vi "Inficon VGC.vi"() -> ()   [LabVIEW 2015]
doc: "Example VI that demonstrates all library features."
uses:
  PL Inficon VGC.lvclass
panel:
  in  "error acknowledgement":u16(ring) items=["manual", "auto"]
  out "temperature, °C":i32
  in  "Torr lock":u16(ring) items=["off", "on"]
  in  "test keys":bool
  out "relay test relays":bool[](array[boolean])
  out "relay test state":u16(ring) items=["off", "on"]
  in  "test relays":bool
  in  "test flash":bool
  in  "test EEPROM":bool
  in  "usb flash inserted":bool
  in  "test display":bool
  in  "test ID resistance":bool
  in  "test ADC":bool
  out "operating hours":u32
  out "MAC address":string
  in  "keylock":u16(ring) items=["off", "on"]
  in  "compatibility":u16(ring) items=["Inficon gauges", "OLV transmitter"]
  in  "usb":T1 {"state" items=["loaded", "loading", "load", "format", "delete"]}
  in  "data logger":T2 {"decimal separator" items=["comma", "point"]; "interval" items=["1 s", "10 s", "30 s", "60 s", "value change >= 1 %", "value change >= 5 %"]; "action" items=["stop", "start", "clear"]}
  in  "date and time":timestamp
  out "device information":T3
  in  "parameters":u16(ring) items=["default", "user"]
  in  "save parameters":bool
  in  "pressure unit":u16(ring)=4 items=["mbar/bar", "Torr", "Pa", "uHg", "hPa", "V"]
  in  "Pirani range\nextension":u16(ring) items=["disabled", "enabled"]
  in  "error relay":u16(ring) items=["all", "unit", "sensor 1 & unit", "sensor 2 & unit", "sensor 3 & unit"]
  in  "display settings":T4 {"bar graph"."graph mode" items=["off", "full scale", "full scale, high level", "full scale, setpoint", "decade", "decade, high level", "decade setpoint", "f(t), 0.2 s/pixel", "f(t), 1 s/pixel", "f(t), 6 s/pixel", "f(t), 1 min./pixel"]; "bar graph"."channel" items=["channel 1", "channel 2", "channel 3"]; "display resolutions" items=["auto", "1 digit", "2 digits", "3 digits", "4 digits"]; "range" items=["UR/OR", "value"]; "number format" items=["floating point", "exponential"]; "language" items=["English", "German", "French"]; "screensaver" items=["off", "10 min.", "30 min.", "1 hour", "2 hours", "8 hours", "backlight off after 1 min."]; "contrast, %" scale=0.0..100.0; "backlight, %" scale=0.0..100.0}
  in  "communication settings":T5={"baud rate"=115200, "ethernet"={"dhcp"=0, "ip address"="", "subnet mask"="", "default gateway"=""}} {"ethernet"."dhcp" items=["disabled", "enabled"]; "baud rate" items=["9600"=9600, "19200"=19200, "38400"=38400, "57600"=57600, "115200"=115200]}
  in  "analog output":cluster{"channel":u16, "characteristic":u16} {"characteristic" items=["log", "log a", "log -6", "log -3", "log +0", "log +3", "log c1", "log c2", "log c3", "lin -10", "lin -9", "lin -8", "lin -7", "lin -6", "lin -5", "lin -4", "lin -3", "lin -2", "lin -1", "lin +0", "lin +1", "lin +2", "lin +3", "IM221", "log c4", "PM411", "ch x", "PRM10K", "IMR110", "IMR120", "IMR310", "IMR320"]; "channel" items=["channel 1", "channel 2", "channel 3"]}
  in  "gauge activation":T6 {"deactivation" items=["manual"=0, "self control"=1, "channel 1"=3, "channel 2"=4, "channel 3"=5]; "thresholds"."off" format="%#_5p"; "thresholds"."on" format="%#_5p"; "activation" items=["manual"=0, "hot start"=1, "channel 1"=3, "channel 2"=4, "channel 3"=5]}
  in  "gauge index":u16(ring)=1 caption="gauge" items=["1"=1, "2"=2, "3"=3]
  in  "continuous time interval":u16(ring)=1 items=["100 ms", "1 s", "1 min."]
  out "continuous read":bool
  out "continuous measurement graph":cluster{dbl, dbl, dbl[][]}(graph)
  in  "continuous measurement":bool
  in  "reset errors":bool
  in  "offset values":dbl[](array[numeric])
  in  "offset modes":u16[](array[ring]) items=["off", "on", "auto", "zero"]
  in  "HV":u16[](array[ring]) items=["off", "on"]
  in  "gas correction":u16[](array[ring]) items=["nitrogen/air", "argon", "hydrogen", "helium", "neon", "krypton", "xenon", "other"]
  in  "ranges":u16[](array[ring]) items=["0.01 mbar", "0.01 Torr", "0.02 mbar", "0.02 Torr", "0.05 mbar", "0.05 Torr", "0.1 mbar", "0.1 Torr", "0.25 mbar", "0.25 Torr", "0.5 mbar", "0.5 Torr", "1 mbar", "1 Torr", "2 mbar", "2 Torr", "5 mbar", "5 Torr", "10 mbar", "10 Torr", "20 mbar", "20 Torr", "50 mbar", "50 Torr", "100 mbar", "100 Torr", "200 mbar", "200 Torr", "500 mbar", "500 Torr", "1000 mbar", "1100 mbar", "1000 Torr", "2 bar", "5 bar", "10 bar", "50 bar"]
  in  "filters":u16[](array[ring]) items=["off", "fast", "normal", "slow"]
  in  "filaments":u16[](array[ring]) items=["auto", "filament 1", "filament 2"]
  in  "emissions":u16[](array[ring]) items=["manual", "auto"]
  in  "degas":u16[](array[ring]) items=["off", "on"]
  in  "calibration factors":dbl[](array[numeric]) format="%#.3g"
  in  "switching function index":u16(ring)=1 caption="switching function" items=["1"=1, "2"=2, "3"=3, "4"=4, "5"=5, "6"=6]
  in  "switching function":T7={"mode"=1, "thresholds"={"lower"=0.0, "upper"=0.0}, "on"=FALSE} {"thresholds"."upper" format="%#_5p"; "thresholds"."lower" format="%#_5p"; "mode" items=["off", "on", "channel 1", "channel 2", "channel 3"]}
  out "gauges":T8(array[cluster]) {"status" items=["data ok", "underrange", "overrange", "sensor error", "sensor off", "no sensor", "identification error", "error BPG, HPG, BCG"]; "value" format="%#_4p"}
  out "combined measured value":dbl
  in  "combined measurement channels":u16[](array[ring]) items=["no gauge", "channel 1", "channel 2", "channel 3"]
  out "error status":T9
  out "VGC":refnum<class "PL Inficon VGC.lvclass">
  in  "interface":enum32{"serial", "TCP"}(tab)
  in  "serial settings":T10={"port"="", "baud rate"=115200} {"baud rate" items=["9600"=9600, "19200"=19200, "38400"=38400, "57600"=57600, "115200"=115200]}
  in  "TCP settings":cluster{"ip address":string, "port":u16}={"ip address"="192.168.1.1", "port"=8000}
  out "error":errorcluster
  in  "stop":bool
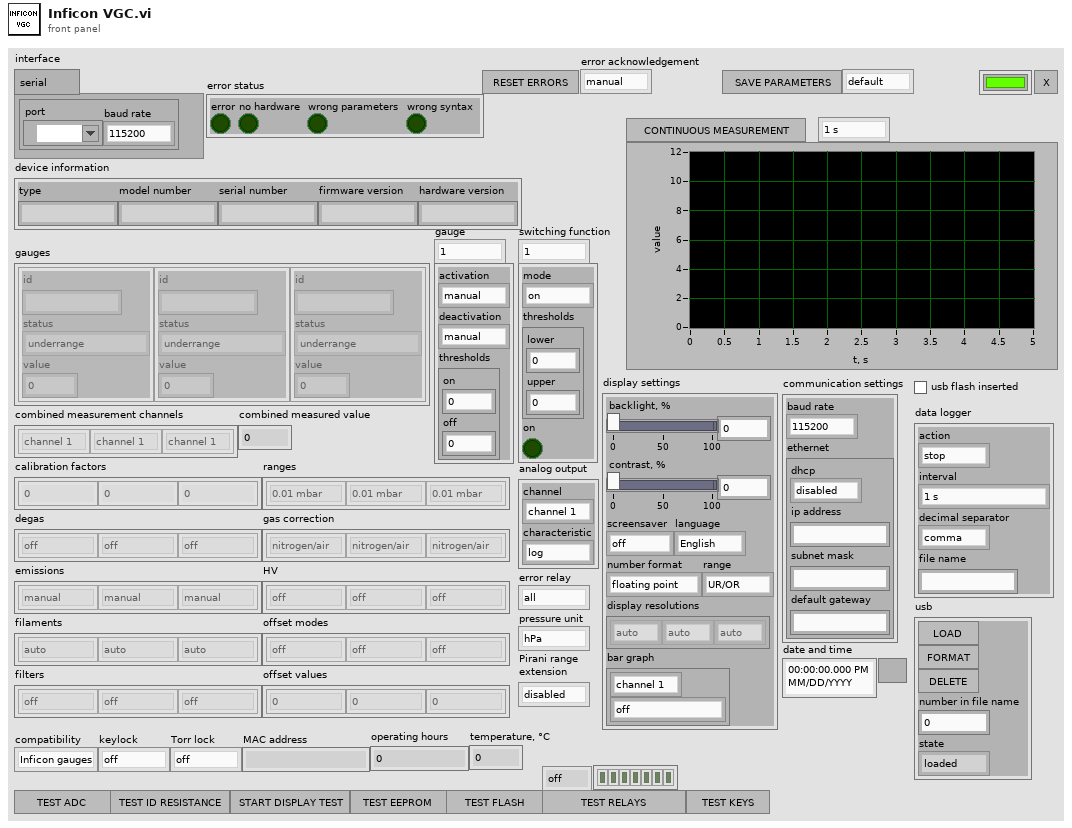
[diagram p1: front panel]
types:
  T1 = cluster{"load":bool, "format":bool, "delete":bool, "number in file name":u8, "state":u16}
  T2 = cluster{"action":u16, "interval":u16, "decimal separator":u16, "file name":string}
  T3 = cluster{"type":string, "model number":string, "serial number":string, "firmware version":string, "hardware version":string}
  T4 = cluster{"backlight, %":u8, "contrast, %":u8, "screensaver":u16, "language":u16, "number format":u16, "range":u16, "display resolutions":u16[], "bar graph":cluster{"channel":u16, "graph mode":u16}}
  T5 = cluster{"baud rate":u32, "ethernet":cluster{"dhcp":u32, "ip address":string, "subnet mask":string, "default gateway":string}}
  T6 = cluster{"activation":u16, "deactivation":u16, "thresholds":cluster{"on":dbl, "off":dbl}}
  T7 = cluster{"mode":u16, "thresholds":cluster{"lower":dbl, "upper":dbl}, "on":bool}
  T8 = cluster{"id":string, "status":u16, "value":dbl}[]
  T9 = cluster{"error":bool, "no hardware":bool, "wrong parameters":bool, "wrong syntax":bool}
  T10 = cluster{"port":refnum<visa-resource-name>, "baud rate":u32}
  T11 = cluster{"switching function relay 1":bool, "switching function relay 2":bool, "switching function relay 3":bool, "switching function relay 4":bool, "switching function relay 5":bool, "switching function relay 6":bool, "error relay":bool}
  T12 = cluster{"String":string, "status":u16, "value":dbl}
  T13 = cluster{"Boolean array[0]":bool, "Boolean array[1]":bool, "Boolean array[2]":bool, "Boolean array[3]":bool, "Boolean array[4]":bool, "Boolean array[5]":bool, "Boolean array[6]":bool}
  T14 = cluster{"key 1":u16, "key 2":u16, "key 3":u16, "key 4":u16}
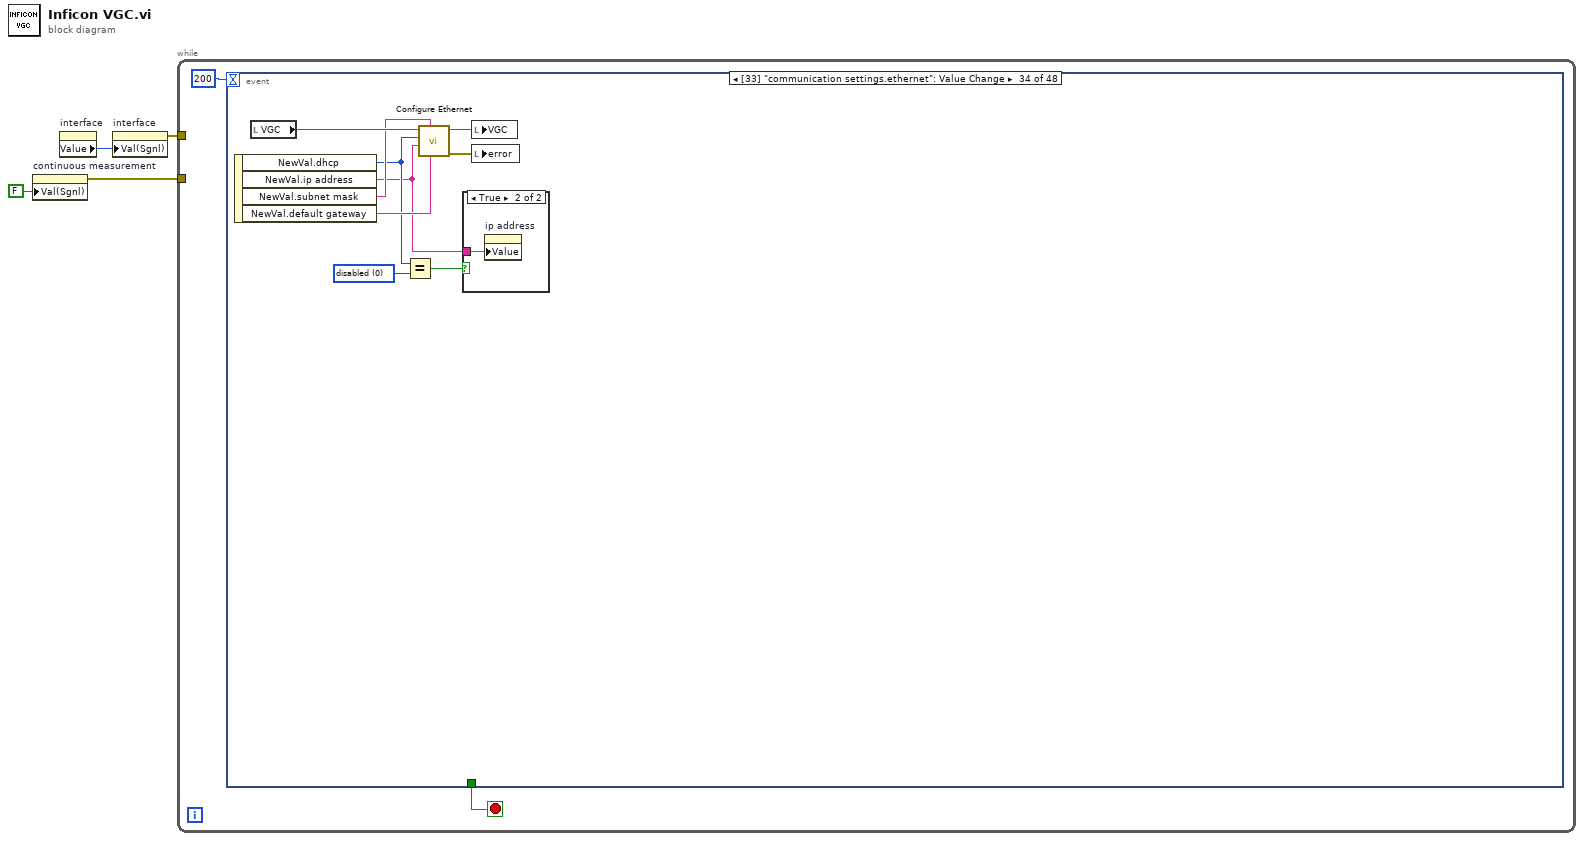
[diagram p0: block diagram]
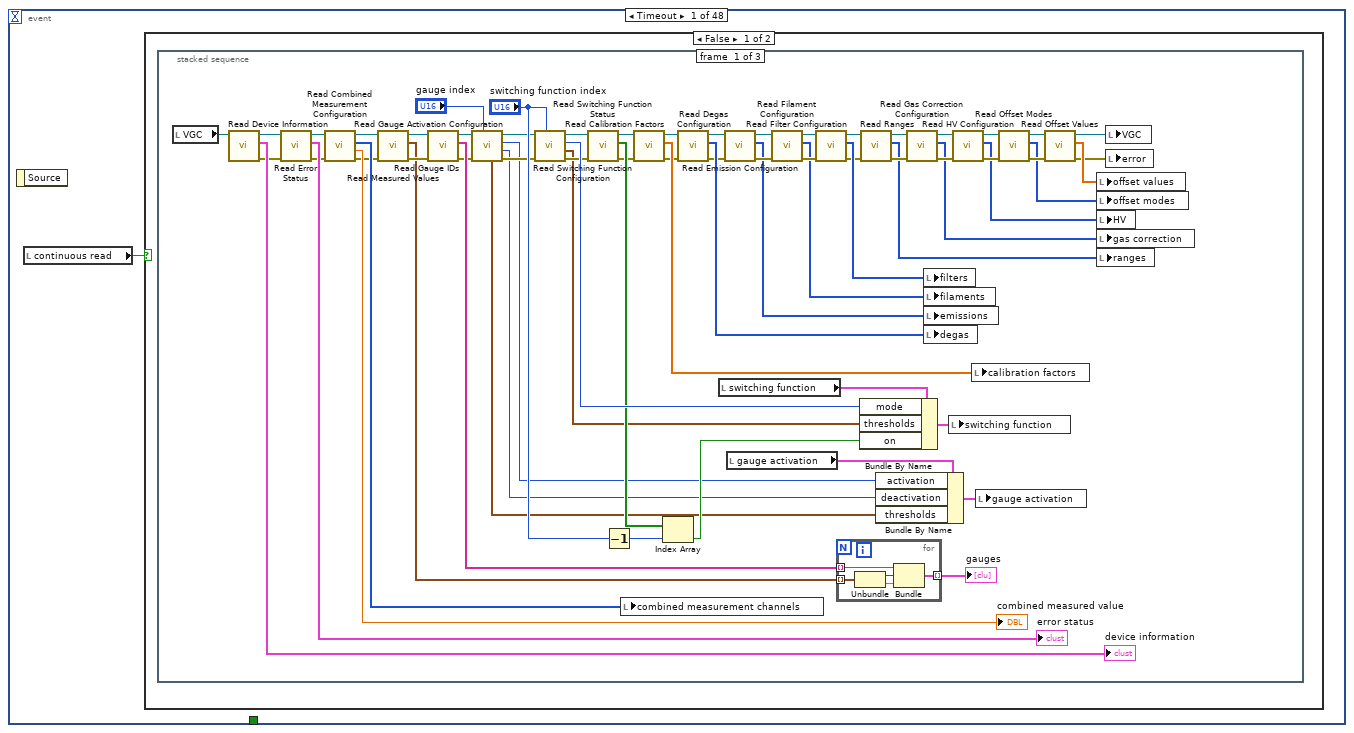
[diagram p2: hidden frame]
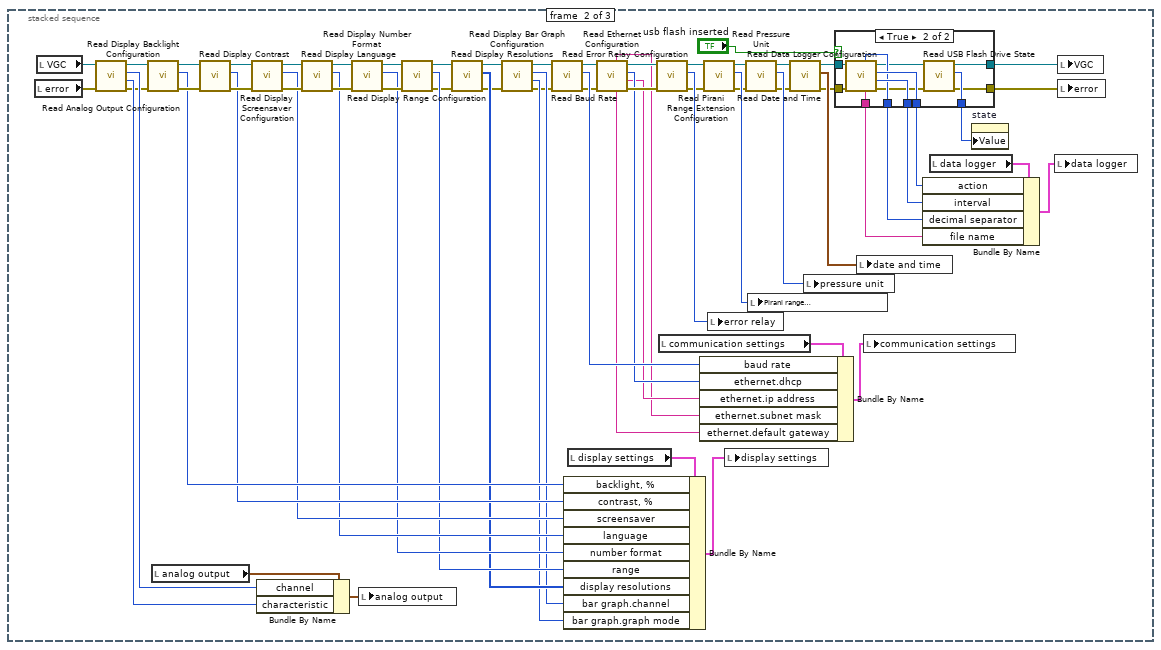
[diagram p3: hidden frame]
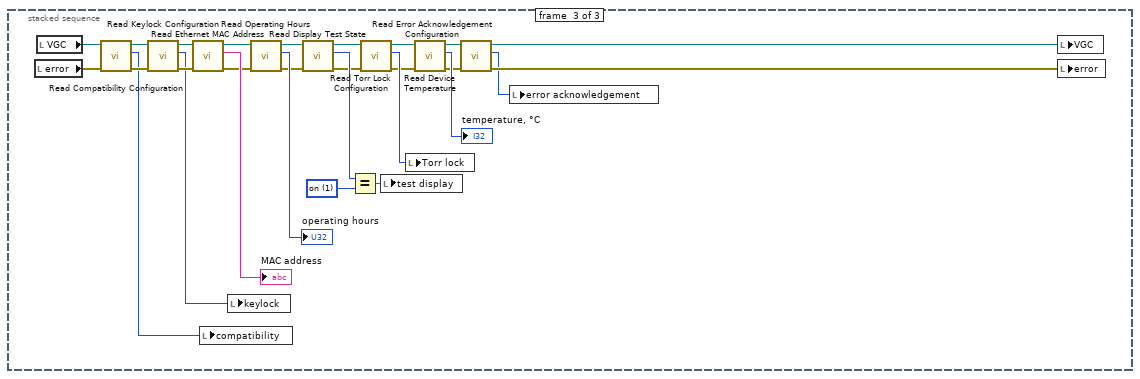
[diagram p5: hidden frame]
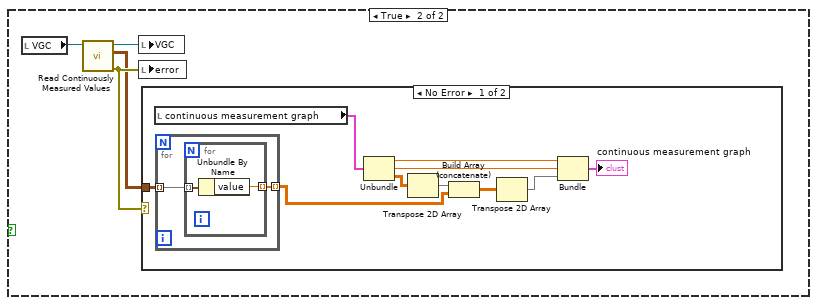
[diagram p6: hidden frame]
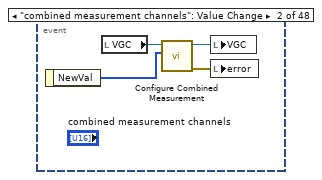
[diagram p8: hidden frame]
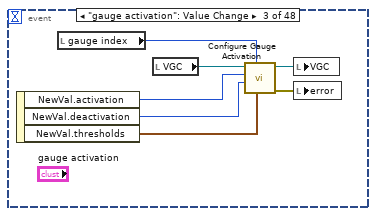
[diagram p9: hidden frame]
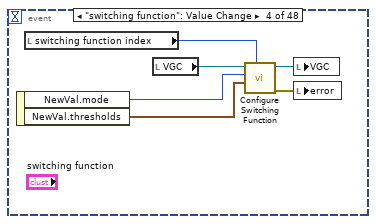
[diagram p10: hidden frame]
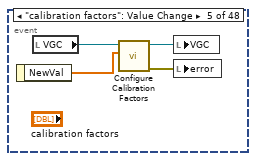
[diagram p11: hidden frame]
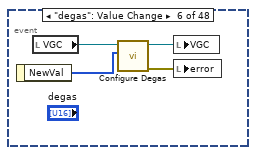
[diagram p12: hidden frame]
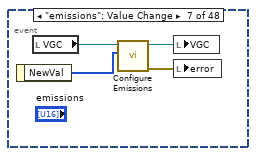
[diagram p13: hidden frame]
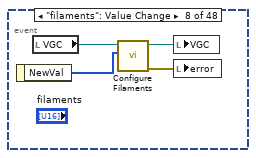
[diagram p14: hidden frame]
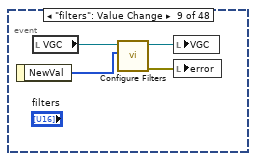
[diagram p15: hidden frame]
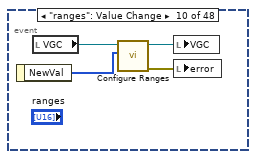
[diagram p16: hidden frame]
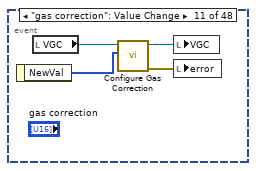
[diagram p17: hidden frame]
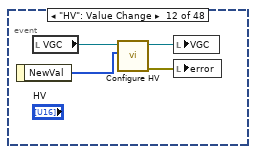
[diagram p18: hidden frame]
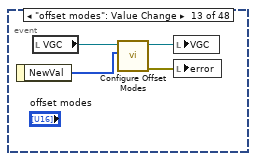
[diagram p19: hidden frame]
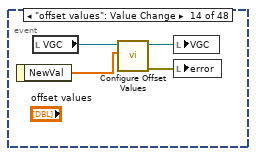
[diagram p20: hidden frame]
diagram:
  n1 = property on="continuous measurement" class="Bool (strict)"("Val(Sgnl)"=FALSE ("Value (Signaling)")) -> (error out=w1:errorcluster)  [unwired: 2 in, 1 out]
  n2 = property on="interface" class="TabCtl (strict)"() -> ("Value"=w4:enum32{"serial", "TCP"})  [unwired: 2 in, 2 out]
  n3 = property on="interface" class="TabCtl (strict)"("Val(Sgnl)"=w4) -> (error out=w3:errorcluster)  [unwired: 2 in, 1 out]
  n4 = while {
    tunnel: w3 -> [_]
    tunnel: w1 -> [_]
    stop <- w5 stop-if-true
    n5 = event shown="[33] \"communication settings.ethernet\": Value Change" {
      selector: _ -> [_ _ _ _ _ _ _ _ _ _ _ _ _ _ _ _ _ _ _ _ _ _ _ _ _ _ _ _ _ _ _ _ _ _ _ _ _ _ _ _ _ _ _ _ _ _ _ _]
      dyn-events: _ -> [_ _ _ _ _ _ _ _ _ _ _ _ _ _ _ _ _ _ _ _ _ _ _ _ _ _ _ _ _ _ _ _ _ _ _ _ _ _ _ _ _ _ _ _ _ _ _ _]
      timeout: 200 -> [_ _ _ _ _ _ _ _ _ _ _ _ _ _ _ _ _ _ _ _ _ _ _ _ _ _ _ _ _ _ _ _ _ _ _ _ _ _ _ _ _ _ _ _ _ _ _ _]
      tunnel: [_ _ _ _ _ _ _ _ _ _ _ _ _ _ _ _ _ _ _ _ _ _ _ _ _ _ _ _ _ _ _ _ _ _ _ _ _ _ _ _ _ _ _ _ _ _ _ TRUE ("stop")] -> w5
      event Timeout {
        n6 = event-data() -> ()  [unwired: 1 in, 1 out]
        n7 = local read "continuous read"() -> (w7:bool)
        n8 = case shown="False" w7 {
          frame False {
            n9 = stacked-sequence {
              frame #0 {
                n10 = local read "VGC"() -> (w11:refnum<class "PL Inficon VGC.lvclass">)
                n11 = call "Read Device Information.vi"("VGC in"=w11) -> ("error out"=w8:errorcluster, "information"=→"device information":T3, "VGC out"=w9:refnum<class "PL Inficon VGC.lvclass">)  [unwired: 8 in]
                n12 = call "Read Error Status.vi"("error in (no error)"=w8, "VGC in"=w9) -> ("error out"=w71:errorcluster, "error status"=→"error status":T9, "VGC out"=w74:refnum<class "PL Inficon VGC.lvclass">)  [unwired: 7 in]
                n13 = call "Read Combined Measurement Configuration.vi"("error in (no error)"=w71, "VGC in"=w74) -> ("error out"=w69:errorcluster, "measured value"=→"combined measured value":dbl, "channels"=w72:u16[], "VGC out"=w70:refnum<class "PL Inficon VGC.lvclass">)  [unwired: 6 in]
                n14 = call "Read Measured Values.vi"("error in (no error)"=w69, "VGC in"=w70) -> ("error out"=w67:errorcluster, "measured values"=w65:cluster{"status":u16, "value":dbl}[], "VGC out"=w68:refnum<class "PL Inficon VGC.lvclass">)  [unwired: 7 in]
                n15 = call "Read Gauge IDs.vi"("error in (no error)"=w67, "VGC in"=w68) -> ("error out"=w22:errorcluster, "gauge ids"=w66:string[], "VGC out"=w25:refnum<class "PL Inficon VGC.lvclass">)  [unwired: 7 in]
                n16 = call "Read Gauge Activation Configuration.vi"("gauge"="gauge index", "error in (no error)"=w22, "VGC in"=w25) -> ("error out"=w23:errorcluster, "deactivation"=w17:u16, "activation"=w18:u16, "VGC out"=w24:refnum<class "PL Inficon VGC.lvclass">, "thresholds"=w16:cluster{"on":dbl, "off":dbl})  [unwired: 4 in]
                n17 = call "Read Switching Function Configuration.vi"("function"="switching function index", "error in (no error)"=w23, "VGC in"=w24) -> ("error out"=w60:errorcluster, "thresholds"=w26:cluster{"lower":dbl, "upper":dbl}, "mode"=w62:u16, "VGC out"=w61:refnum<class "PL Inficon VGC.lvclass">)  [unwired: 5 in]
                n18 = call "Read Switching Function Status.vi"("error in (no error)"=w60, "VGC in"=w61) -> ("error out"=w55:errorcluster, "status"=w59:bool[], "VGC out"=w54:refnum<class "PL Inficon VGC.lvclass">)  [unwired: 7 in]
                n19 = Decrement(x="switching function index") -> (x-1=w58:u16)
                n20 = local write "combined measurement channels"(w72) -> ()
                n21 = call "Read Calibration Factors.vi"("error in (no error)"=w55, "VGC in"=w54) -> ("error out"=w12:errorcluster, "calibration factors"=w53:dbl[], "VGC out"=w13:refnum<class "PL Inficon VGC.lvclass">)  [unwired: 7 in]
                n22 = Index Array(array=w59, index=w58) -> (element=w57:bool)
                n23 = call "Read Degas Configuration.vi"("error in (no error)"=w12, "VGC in"=w13) -> ("error out"=w51:errorcluster, "degas"=w52:u16[], "VGC out"=w46:refnum<class "PL Inficon VGC.lvclass">)  [unwired: 7 in]
                n24 = local read "switching function"() -> (w63:T7)
                n25 = call "Read Emission Configuration.vi"("error in (no error)"=w51, "VGC in"=w46) -> ("error out"=w50:errorcluster, "emissions"=w45:u16[], "VGC out"=w47:refnum<class "PL Inficon VGC.lvclass">)  [unwired: 7 in]
                n26 = local read "gauge activation"() -> (w20:T6)
                n27 = call "Read Filament Configuration.vi"("error in (no error)"=w50, "VGC in"=w47) -> ("error out"=w49:errorcluster, "filaments"=w44:u16[], "VGC out"=w48:refnum<class "PL Inficon VGC.lvclass">)  [unwired: 7 in]
                n28 = call "Read Filter Configuration.vi"("error in (no error)"=w49, "VGC in"=w48) -> ("error out"=w37:errorcluster, "filters"=w43:u16[], "VGC out"=w42:refnum<class "PL Inficon VGC.lvclass">)  [unwired: 7 in]
                n29 = for {
                  tunnel: w66 -> [w79] mode=indexing
                  tunnel: w65 -> [w80] mode=indexing
                  tunnel: [w76] -> w64 mode=indexing
                  n30 = Unbundle(w80) -> ("status"=w78:u16, "value"=w77:dbl)
                  n31 = Bundle("String"=w79, "status"=w78, "value"=w77) -> (w76:T12)  [unwired: 1 in]
                }
                "gauges" <- w64
                n32 = Bundle By Name(cluster=w63, "mode"=w62, "thresholds"=w26, "on"=w57) -> (w56:T7)
                n33 = call "Read Ranges.vi"("error in (no error)"=w37, "VGC in"=w42) -> ("error out"=w38:errorcluster, "ranges"=w32:u16[], "VGC out"=w41:refnum<class "PL Inficon VGC.lvclass">)  [unwired: 7 in]
                n34 = Bundle By Name(cluster=w20, "activation"=w18, "deactivation"=w17, "thresholds"=w16) -> (w19:T6)
                n35 = call "Read Gas Correction Configuration.vi"("error in (no error)"=w38, "VGC in"=w41) -> ("error out"=w39:errorcluster, "gas correction"=w31:u16[], "VGC out"=w40:refnum<class "PL Inficon VGC.lvclass">)  [unwired: 7 in]
                n36 = local write "filters"(w43) -> ()
                n37 = local write "filaments"(w44) -> ()
                n38 = local write "emissions"(w45) -> ()
                n39 = local write "degas"(w52) -> ()
                n40 = local write "switching function"(w56) -> ()
                n41 = call "Read HV Configuration.vi"("error in (no error)"=w39, "VGC in"=w40) -> ("error out"=w36:errorcluster, "HV"=w30:u16[], "VGC out"=w33:refnum<class "PL Inficon VGC.lvclass">)  [unwired: 7 in]
                n42 = local write "calibration factors"(w53) -> ()
                n43 = local write "gauge activation"(w19) -> ()
                n44 = call "Read Offset Modes.vi"("error in (no error)"=w36, "VGC in"=w33) -> ("error out"=w35:errorcluster, "modes"=w29:u16[], "VGC out"=w34:refnum<class "PL Inficon VGC.lvclass">)  [unwired: 7 in]
                n45 = call "Read Offset Values.vi"("error in (no error)"=w35, "VGC in"=w34) -> ("error out"=w14:errorcluster, "values"=w28:dbl[], "VGC out"=w15:refnum<class "PL Inficon VGC.lvclass">)  [unwired: 7 in]
                n46 = local write "offset values"(w28) -> ()
                n47 = local write "offset modes"(w29) -> ()
                n48 = local write "HV"(w30) -> ()
                n49 = local write "gas correction"(w31) -> ()
                n50 = local write "ranges"(w32) -> ()
                n51 = local write "VGC"(w15) -> ()
                n52 = local write "error"(w14) -> ()
              }
              frame #1 {
                n53 = local read "error"() -> (w141:errorcluster)
                n54 = local read "VGC"() -> (w143:refnum<class "PL Inficon VGC.lvclass">)
                n55 = call "Read Analog Output Configuration.vi"("error in (no error)"=w141, "VGC in"=w143) -> ("error out"=w144:errorcluster, "characteristic"=w147:u16, "channel"=w148:u16, "VGC out"=w145:refnum<class "PL Inficon VGC.lvclass">)  [unwired: 6 in]
                n56 = call "Read Display Backlight Configuration.vi"("error in (no error)"=w144, "VGC in"=w145) -> ("error out"=w137:errorcluster, "backlight, %"=w130:u8, "VGC out"=w138:refnum<class "PL Inficon VGC.lvclass">)  [unwired: 7 in]
                n57 = local read "analog output"() -> (w142:cluster{"channel":u16, "characteristic":u16})
                n58 = call "Read Display Contrast.vi"("error in (no error)"=w137, "VGC in"=w138) -> ("error out"=w135:errorcluster, "contrast, %"=w129:u8, "VGC out"=w136:refnum<class "PL Inficon VGC.lvclass">)  [unwired: 7 in]
                n59 = call "Read Display Screensaver Configuration.vi"("error in (no error)"=w135, "VGC in"=w136) -> ("error out"=w134:errorcluster, "screensaver"=w126:u16, "VGC out"=w132:refnum<class "PL Inficon VGC.lvclass">)  [unwired: 7 in]
                n60 = Bundle By Name(cluster=w142, "channel"=w148, "characteristic"=w147) -> (w146:cluster{"channel":u16, "characteristic":u16})
                n61 = call "Read Display Language.vi"("error in (no error)"=w134, "VGC in"=w132) -> ("error out"=w133:errorcluster, "language"=w125:u16, "VGC out"=w131:refnum<class "PL Inficon VGC.lvclass">)  [unwired: 7 in]
                n62 = call "Read Display Number Format.vi"("error in (no error)"=w133, "VGC in"=w131) -> ("error out"=w127:errorcluster, "format"=w124:u16, "VGC out"=w128:refnum<class "PL Inficon VGC.lvclass">)  [unwired: 7 in]
                n63 = local write "analog output"(w146) -> ()
                n64 = call "Read Display Range Configuration.vi"("error in (no error)"=w127, "VGC in"=w128) -> ("error out"=w98:errorcluster, "mode"=w123:u16, "VGC out"=w117:refnum<class "PL Inficon VGC.lvclass">)  [unwired: 7 in]
                n65 = call "Read Display Resolutions.vi"("error in (no error)"=w98, "VGC in"=w117) -> ("error out"=w97:errorcluster, "display resolutions"=w122:u16[], "VGC out"=w116:refnum<class "PL Inficon VGC.lvclass">)  [unwired: 7 in]
                n66 = call "Read Display Bar Graph Configuration.vi"("error in (no error)"=w97, "VGC in"=w116) -> ("error out"=w118:errorcluster, "graph mode"=w120:u16, "channel"=w121:u16, "VGC out"=w119:refnum<class "PL Inficon VGC.lvclass">)  [unwired: 6 in]
                n67 = call "Read Baud Rate.vi"("error in (no error)"=w118, "VGC in"=w119) -> ("error out"=w105:errorcluster, "baud rate"=w113:u32, "VGC out"=w106:refnum<class "PL Inficon VGC.lvclass">)  [unwired: 7 in]
                n68 = local read "display settings"() -> (w140:T4)
                n69 = Bundle By Name(cluster=w140, "backlight, %"=w130, "contrast, %"=w129, "screensaver"=w126, "language"=w125, "number format"=w124, "range"=w123, "display resolutions"=w122, "bar graph.channel"=w121, "bar graph.graph mode"=w120) -> (w139:T4)
                n70 = call "Read Ethernet Configuration.vi"("error in (no error)"=w105, "VGC in"=w106) -> ("error out"=w104:errorcluster, "ip address"=w101:string, "dhcp"=w102:u32, "VGC out"=w103:refnum<class "PL Inficon VGC.lvclass">, "default gateway"=w99:string, "subnet mask"=w100:string)  [unwired: 4 in]
                n71 = call "Read Error Relay Configuration.vi"("error in (no error)"=w104, "VGC in"=w103) -> ("error out"=w107:errorcluster, "errors"=w112:u16, "VGC out"=w111:refnum<class "PL Inficon VGC.lvclass">)  [unwired: 7 in]
                n72 = local read "communication settings"() -> (w115:T5)
                n73 = Bundle By Name(cluster=w115, "baud rate"=w113, "ethernet.dhcp"=w102, "ethernet.ip address"=w101, "ethernet.subnet mask"=w100, "ethernet.default gateway"=w99) -> (w114:T5)
                n74 = call "Read Pirani Range Extension Configuration.vi"("error in (no error)"=w107, "VGC in"=w111) -> ("error out"=w108:errorcluster, "range extension"=w110:u16, "VGC out"=w109:refnum<class "PL Inficon VGC.lvclass">)  [unwired: 7 in]
                n75 = local write "error relay"(w112) -> ()
                n76 = local write "display settings"(w139) -> ()
                n77 = call "Read Pressure Unit.vi"("error in (no error)"=w108, "VGC in"=w109) -> ("error out"=w94:errorcluster, "unit"=w96:u16, "VGC out"=w95:refnum<class "PL Inficon VGC.lvclass">)  [unwired: 7 in]
                n78 = local write "Pirani range\nextension"(w110) -> ()
                n79 = call "Read Date and Time.vi"("error in (no error)"=w94, "VGC in"=w95) -> ("error out"=w91:errorcluster, "date and time"=w93:timestamp, "VGC out"=w92:refnum<class "PL Inficon VGC.lvclass">)  [unwired: 7 in]
                n80 = local write "pressure unit"(w96) -> ()
                n81 = case shown="True" "usb flash inserted" {
                  tunnel: w92 -> [w150 w161]
                  tunnel: w91 -> [w149 w160]
                  tunnel: [_ w159] -> w88
                  tunnel: [_ w158] -> w87
                  tunnel: [_ w157] -> w86
                  tunnel: [_ w156] -> w85
                  tunnel: [_ w153] -> w84
                  tunnel: [w149 w152] -> w83
                  tunnel: [w150 w151] -> w82
                  frame False {
                  }
                  frame True {
                    n82 = call "Read Data Logger Configuration.vi"("error in (no error)"=w160, "VGC in"=w161) -> ("error out"=w154:errorcluster, "interval"=w158:u16, "action"=w159:u16, "VGC out"=w155:refnum<class "PL Inficon VGC.lvclass">, "file name"=w156:string, "decimal separator"=w157:u16)  [unwired: 4 in]
                    n83 = call "Read USB Flash Drive State.vi"("error in (no error)"=w154, "VGC in"=w155) -> ("error out"=w152:errorcluster, "state"=w153:u16, "VGC out"=w151:refnum<class "PL Inficon VGC.lvclass">)  [unwired: 7 in]
                  }
                }
                n84 = local write "date and time"(w93) -> ()
                n85 = local write "communication settings"(w114) -> ()
                n86 = local read "data logger"() -> (w89:T2)
                n87 = Bundle By Name(cluster=w89, "action"=w88, "interval"=w87, "decimal separator"=w86, "file name"=w85) -> (w90:T2)
                n88 = property on="state" class="Ring (strict)"("Value"=w84) -> ()  [unwired: 2 in, 2 out]
                n89 = local write "data logger"(w90) -> ()
                n90 = local write "VGC"(w82) -> ()
                n91 = local write "error"(w83) -> ()
              }
              frame #2 {
                w174 = u16 1 items=["off", "on"] ("display test state")
                n92 = local read "error"() -> (w188:errorcluster)
                n93 = local read "VGC"() -> (w189:refnum<class "PL Inficon VGC.lvclass">)
                n94 = call "Read Compatibility Configuration.vi"("error in (no error)"=w188, "VGC in"=w189) -> ("error out"=w186:errorcluster, "compatibility"=w182:u16, "VGC out"=w187:refnum<class "PL Inficon VGC.lvclass">)  [unwired: 7 in]
                n95 = call "Read Keylock Configuration.vi"("error in (no error)"=w186, "VGC in"=w187) -> ("error out"=w185:errorcluster, "keylock"=w181:u16, "VGC out"=w184:refnum<class "PL Inficon VGC.lvclass">)  [unwired: 7 in]
                n96 = call "Read Ethernet MAC Address.vi"("error in (no error)"=w185, "VGC in"=w184) -> ("error out"=w179:errorcluster, "MAC address"=→"MAC address":string, "VGC out"=w180:refnum<class "PL Inficon VGC.lvclass">)  [unwired: 7 in]
                n97 = local write "compatibility"(w182) -> ()
                n98 = local write "keylock"(w181) -> ()
                n99 = call "Read Operating Hours.vi"("error in (no error)"=w179, "VGC in"=w180) -> ("error out"=w176:errorcluster, "operating hours"=→"operating hours":u32, "VGC out"=w177:refnum<class "PL Inficon VGC.lvclass">)  [unwired: 7 in]
                n100 = call "Read Display Test State.vi"("error in (no error)"=w176, "VGC in"=w177) -> ("error out"=w171:errorcluster, "display test state"=w175:u16, "VGC out"=w172:refnum<class "PL Inficon VGC.lvclass">)  [unwired: 7 in]
                n101 = Equal?(x=w175, y=w174) -> (x = y?=w173:bool)
                n102 = call "Read Torr Lock Configuration.vi"("error in (no error)"=w171, "VGC in"=w172) -> ("error out"=w169:errorcluster, "Torr lock"=w170:u16, "VGC out"=w168:refnum<class "PL Inficon VGC.lvclass">)  [unwired: 7 in]
                n103 = local write "test display"(w173) -> ()
                n104 = local write "Torr lock"(w170) -> ()
                n105 = call "Read Device Temperature.vi"("error in (no error)"=w169, "VGC in"=w168) -> ("error out"=w165:errorcluster, "temperature, °C"=→"temperature, °C":i32, "VGC out"=w166:refnum<class "PL Inficon VGC.lvclass">)  [unwired: 7 in]
                n106 = call "Read Error Acknowledgement Configuration.vi"("error in (no error)"=w165, "VGC in"=w166) -> ("error out"=w164:errorcluster, "error acknowledgement"=w162:u16, "VGC out"=w163:refnum<class "PL Inficon VGC.lvclass">)  [unwired: 7 in]
                n107 = local write "error acknowledgement"(w162) -> ()
                n108 = local write "VGC"(w163) -> ()
                n109 = local write "error"(w164) -> ()
              }
            }
          }
          frame True {
            n110 = local read "VGC"() -> (w193:refnum<class "PL Inficon VGC.lvclass">)
            n111 = call "Read Continuously Measured Values.vi"("VGC in"=w193) -> ("error out"=w191:errorcluster, "measured values"=w190:cluster{"status":u16, "value":dbl}[][], "VGC out"=w192:refnum<class "PL Inficon VGC.lvclass">)  [unwired: 8 in]
            n112 = local write "VGC"(w192) -> ()
            n113 = local write "error"(w191) -> ()
            n114 = case shown="No Error" w191 {
              tunnel: w190 -> [w203 _]
              frame No Error {
                n115 = local read "continuous measurement graph"() -> (w202:cluster{dbl, dbl, dbl[][]})
                n116 = for {
                  tunnel: w203 -> [w205] mode=indexing
                  tunnel: [w204] -> w194 mode=indexing
                  n117 = for {
                    tunnel: w205 -> [w207] mode=indexing
                    tunnel: [w206] -> w204 mode=indexing
                    n118 = Unbundle By Name(w207) -> ("value"=w206:dbl)
                  }
                }
                n119 = Unbundle(w202) -> (w201:dbl, w199:dbl, w198:dbl[][])
                n120 = Transpose 2D Array(2D array=w198) -> (transposed array=w197:dbl[][])
                n121 = Build Array (concatenate)(w197, w194) -> (w196:dbl[][])
                n122 = Transpose 2D Array(2D array=w196) -> (transposed array=w195:dbl[][])
                n123 = Bundle(w201, w199, w195) -> (→"continuous measurement graph":cluster{dbl, dbl, dbl[][]})  [unwired: 1 in]
              }
              frame Error {
              }
            }
          }
        }
      }
      event "combined measurement channels": Value Change {
        n124 = event-data() -> ("NewVal"=w208:u16[])  [unwired: 1 in]
        n125 = local read "VGC"() -> (w211:refnum<class "PL Inficon VGC.lvclass">)
        n126 = call "Configure Combined Measurement.vi"("channels"=w208, "VGC in"=w211) -> ("error out"=w209:errorcluster, "VGC out"=w210:refnum<class "PL Inficon VGC.lvclass">)  [unwired: 6 in, 2 out]
        n127 = local write "VGC"(w210) -> ()
        n128 = local write "error"(w209) -> ()
      }
      event "gauge activation": Value Change {
        n129 = event-data() -> ("NewVal.activation"=w214:u16, "NewVal.deactivation"=w213:u16, "NewVal.thresholds"=w212:cluster{"on":dbl, "off":dbl})  [unwired: 1 in]
        n130 = local read "gauge index"() -> (w218:u16)
        n131 = local read "VGC"() -> (w217:refnum<class "PL Inficon VGC.lvclass">)
        n132 = call "Configure Gauge Activation.vi"("thresholds"=w212, "gauge"=w218, "deactivation"=w213, "activation"=w214, "VGC in"=w217) -> ("error out"=w215:errorcluster, "VGC out"=w216:refnum<class "PL Inficon VGC.lvclass">)  [unwired: 2 in, 3 out]
        n133 = local write "VGC"(w216) -> ()
        n134 = local write "error"(w215) -> ()
      }
      event "switching function": Value Change {
        n135 = event-data() -> ("NewVal.mode"=w220:u16, "NewVal.thresholds"=w219:cluster{"lower":dbl, "upper":dbl})  [unwired: 1 in]
        n136 = local read "switching function index"() -> (w221:u16)
        n137 = local read "VGC"() -> (w223:refnum<class "PL Inficon VGC.lvclass">)
        n138 = call "Configure Switching Function.vi"("function"=w221, "thresholds"=w219, "mode"=w220, "VGC in"=w223) -> ("error out"=w222:errorcluster, "VGC out"=w224:refnum<class "PL Inficon VGC.lvclass">)  [unwired: 4 in, 2 out]
        n139 = local write "VGC"(w224) -> ()
        n140 = local write "error"(w222) -> ()
      }
      event "calibration factors": Value Change {
        n141 = event-data() -> ("NewVal"=w225:dbl[])  [unwired: 1 in]
        n142 = local read "VGC"() -> (w226:refnum<class "PL Inficon VGC.lvclass">)
        n143 = call "Configure Calibration Factors.vi"("calibration factors"=w225, "VGC in"=w226) -> ("error out"=w227:errorcluster, "VGC out"=w228:refnum<class "PL Inficon VGC.lvclass">)  [unwired: 7 in, 1 out]
        n144 = local write "VGC"(w228) -> ()
        n145 = local write "error"(w227) -> ()
      }
      event "degas": Value Change {
        n146 = event-data() -> ("NewVal"=w229:u16[])  [unwired: 1 in]
        n147 = local read "VGC"() -> (w230:refnum<class "PL Inficon VGC.lvclass">)
        n148 = call "Configure Degas.vi"("degas"=w229, "VGC in"=w230) -> ("error out"=w231:errorcluster, "VGC out"=w232:refnum<class "PL Inficon VGC.lvclass">)  [unwired: 7 in, 1 out]
        n149 = local write "VGC"(w232) -> ()
        n150 = local write "error"(w231) -> ()
      }
      event "emissions": Value Change {
        n151 = event-data() -> ("NewVal"=w233:u16[])  [unwired: 1 in]
        n152 = local read "VGC"() -> (w234:refnum<class "PL Inficon VGC.lvclass">)
        n153 = call "Configure Emissions.vi"("emissions"=w233, "VGC in"=w234) -> ("error out"=w235:errorcluster, "VGC out"=w236:refnum<class "PL Inficon VGC.lvclass">)  [unwired: 7 in, 1 out]
        n154 = local write "VGC"(w236) -> ()
        n155 = local write "error"(w235) -> ()
      }
      event "filaments": Value Change {
        n156 = event-data() -> ("NewVal"=w237:u16[])  [unwired: 1 in]
        n157 = local read "VGC"() -> (w238:refnum<class "PL Inficon VGC.lvclass">)
        n158 = call "Configure Filaments.vi"("filaments"=w237, "VGC in"=w238) -> ("error out"=w239:errorcluster, "VGC out"=w240:refnum<class "PL Inficon VGC.lvclass">)  [unwired: 7 in, 1 out]
        n159 = local write "VGC"(w240) -> ()
        n160 = local write "error"(w239) -> ()
      }
      event "filters": Value Change {
        n161 = event-data() -> ("NewVal"=w241:u16[])  [unwired: 1 in]
        n162 = local read "VGC"() -> (w242:refnum<class "PL Inficon VGC.lvclass">)
        n163 = call "Configure Filters.vi"("filters"=w241, "VGC in"=w242) -> ("error out"=w243:errorcluster, "VGC out"=w244:refnum<class "PL Inficon VGC.lvclass">)  [unwired: 7 in, 1 out]
        n164 = local write "VGC"(w244) -> ()
        n165 = local write "error"(w243) -> ()
      }
      event "ranges": Value Change {
        n166 = event-data() -> ("NewVal"=w245:u16[])  [unwired: 1 in]
        n167 = local read "VGC"() -> (w246:refnum<class "PL Inficon VGC.lvclass">)
        n168 = call "Configure Ranges.vi"("ranges"=w245, "VGC in"=w246) -> ("error out"=w247:errorcluster, "VGC out"=w248:refnum<class "PL Inficon VGC.lvclass">)  [unwired: 7 in, 1 out]
        n169 = local write "VGC"(w248) -> ()
        n170 = local write "error"(w247) -> ()
      }
      event "gas correction": Value Change {
        n171 = event-data() -> ("NewVal"=w249:u16[])  [unwired: 1 in]
        n172 = local read "VGC"() -> (w250:refnum<class "PL Inficon VGC.lvclass">)
        n173 = call "Configure Gas Correction.vi"("gas correction"=w249, "VGC in"=w250) -> ("error out"=w251:errorcluster, "VGC out"=w252:refnum<class "PL Inficon VGC.lvclass">)  [unwired: 7 in, 1 out]
        n174 = local write "VGC"(w252) -> ()
        n175 = local write "error"(w251) -> ()
      }
      event "HV": Value Change {
        n176 = event-data() -> ("NewVal"=w253:u16[])  [unwired: 1 in]
        n177 = local read "VGC"() -> (w254:refnum<class "PL Inficon VGC.lvclass">)
        n178 = call "Configure HV.vi"("HV"=w253, "VGC in"=w254) -> ("error out"=w255:errorcluster, "VGC out"=w256:refnum<class "PL Inficon VGC.lvclass">)  [unwired: 7 in, 1 out]
        n179 = local write "VGC"(w256) -> ()
        n180 = local write "error"(w255) -> ()
      }
      event "offset modes": Value Change {
        n181 = event-data() -> ("NewVal"=w257:u16[])  [unwired: 1 in]
        n182 = local read "VGC"() -> (w258:refnum<class "PL Inficon VGC.lvclass">)
        n183 = call "Configure Offset Modes.vi"("modes"=w257, "VGC in"=w258) -> ("error out"=w259:errorcluster, "VGC out"=w260:refnum<class "PL Inficon VGC.lvclass">)  [unwired: 7 in, 1 out]
        n184 = local write "VGC"(w260) -> ()
        n185 = local write "error"(w259) -> ()
      }
      event "offset values": Value Change {
        n186 = event-data() -> ("NewVal"=w261:dbl[])  [unwired: 1 in]
        n187 = local read "VGC"() -> (w262:refnum<class "PL Inficon VGC.lvclass">)
        n188 = call "Configure Offset Values.vi"("values"=w261, "VGC in"=w262) -> ("error out"=w263:errorcluster, "VGC out"=w264:refnum<class "PL Inficon VGC.lvclass">)  [unwired: 7 in, 1 out]
        n189 = local write "VGC"(w264) -> ()
        n190 = local write "error"(w263) -> ()
      }
      event "analog output": Value Change {
        n191 = event-data() -> ("NewVal.channel"=w266:u16, "NewVal.characteristic"=w265:u16)  [unwired: 1 in]
        n192 = local read "VGC"() -> (w267:refnum<class "PL Inficon VGC.lvclass">)
        n193 = call "Configure Analog Output.vi"("characteristic"=w265, "channel"=w266, "VGC in"=w267) -> ("error out"=w268:errorcluster, "VGC out"=w269:refnum<class "PL Inficon VGC.lvclass">)  [unwired: 5 in, 2 out]
        n194 = local write "VGC"(w269) -> ()
        n195 = local write "error"(w268) -> ()
      }
      event "error relay": Value Change {
        n196 = event-data() -> ("NewVal"=w270:u16)  [unwired: 1 in]
        n197 = local read "VGC"() -> (w271:refnum<class "PL Inficon VGC.lvclass">)
        n198 = call "Configure Error Relay.vi"("errors"=w270, "VGC in"=w271) -> ("error out"=w272:errorcluster, "VGC out"=w273:refnum<class "PL Inficon VGC.lvclass">)  [unwired: 7 in, 1 out]
        n199 = local write "VGC"(w273) -> ()
        n200 = local write "error"(w272) -> ()
      }
      event "Pirani range\nextension": Value Change {
        n201 = event-data() -> ("NewVal"=w274:u16)  [unwired: 1 in]
        n202 = local read "VGC"() -> (w275:refnum<class "PL Inficon VGC.lvclass">)
        n203 = call "Configure Pirani Range Extension.vi"("range extension"=w274, "VGC in"=w275) -> ("error out"=w276:errorcluster, "VGC out"=w277:refnum<class "PL Inficon VGC.lvclass">)  [unwired: 7 in, 1 out]
        n204 = local write "VGC"(w277) -> ()
        n205 = local write "error"(w276) -> ()
      }
      event "pressure unit": Value Change {
        n206 = event-data() -> ("NewVal"=w278:u16)  [unwired: 1 in]
        n207 = local read "VGC"() -> (w279:refnum<class "PL Inficon VGC.lvclass">)
        n208 = call "Configure Pressure Unit.vi"("unit"=w278, "VGC in"=w279) -> ("error out"=w280:errorcluster, "VGC out"=w281:refnum<class "PL Inficon VGC.lvclass">)  [unwired: 7 in, 1 out]
        n209 = local write "VGC"(w281) -> ()
        n210 = local write "error"(w280) -> ()
      }
      event "date and time": Value Change {
        n211 = event-data() -> ("NewVal"=w282:timestamp)  [unwired: 1 in]
        n212 = local read "VGC"() -> (w283:refnum<class "PL Inficon VGC.lvclass">)
        n213 = call "Configure Date and Time.vi"("date and time"=w282, "VGC in"=w283) -> ("error out"=w284:errorcluster, "VGC out"=w285:refnum<class "PL Inficon VGC.lvclass">)  [unwired: 7 in, 1 out]
        n214 = local write "VGC"(w285) -> ()
        n215 = local write "error"(w284) -> ()
      }
      event "compatibility": Value Change {
        n216 = event-data() -> ("NewVal"=w286:u16)  [unwired: 1 in]
        n217 = local read "VGC"() -> (w287:refnum<class "PL Inficon VGC.lvclass">)
        n218 = call "Configure Compatibility.vi"("compatibility"=w286, "VGC in"=w287) -> ("error out"=w288:errorcluster, "VGC out"=w289:refnum<class "PL Inficon VGC.lvclass">)  [unwired: 7 in, 1 out]
        n219 = local write "VGC"(w289) -> ()
        n220 = local write "error"(w288) -> ()
      }
      event "keylock": Value Change {
        n221 = event-data() -> ("NewVal"=w290:u16)  [unwired: 1 in]
        n222 = local read "VGC"() -> (w291:refnum<class "PL Inficon VGC.lvclass">)
        n223 = call "Configure Keylock.vi"("keylock"=w290, "VGC in"=w291) -> ("error out"=w292:errorcluster, "VGC out"=w293:refnum<class "PL Inficon VGC.lvclass">)  [unwired: 7 in, 1 out]
        n224 = local write "VGC"(w293) -> ()
        n225 = local write "error"(w292) -> ()
      }
      event "Torr lock": Value Change {
        n226 = event-data() -> ("NewVal"=w294:u16)  [unwired: 1 in]
        n227 = local read "VGC"() -> (w295:refnum<class "PL Inficon VGC.lvclass">)
        n228 = call "Configure Torr Lock.vi"("Torr lock"=w294, "VGC in"=w295) -> ("error out"=w296:errorcluster, "VGC out"=w297:refnum<class "PL Inficon VGC.lvclass">)  [unwired: 7 in, 1 out]
        n229 = local write "VGC"(w297) -> ()
        n230 = local write "error"(w296) -> ()
      }
      event "data logger": Value Change {
        n231 = event-data() -> ("NewVal.action"=w301:u16, "NewVal.interval"=w300:u16, "NewVal.decimal separator"=w299:u16, "NewVal.file name"=w298:string)  [unwired: 1 in]
        n232 = local read "VGC"() -> (w302:refnum<class "PL Inficon VGC.lvclass">)
        n233 = call "Configure Data Logger.vi"("file name"=w298, "decimal separator"=w299, "interval"=w300, "action"=w301, "VGC in"=w302) -> ("error out"=w303:errorcluster, "VGC out"=w304:refnum<class "PL Inficon VGC.lvclass">)  [unwired: 1 in, 4 out]
        n234 = local write "VGC"(w304) -> ()
        n235 = local write "error"(w303) -> ()
      }
      event "usb.load", "usb.format", "usb.delete": Value Change {
        w307 = u16 2 items=["load"=2, "format"=3, "delete"=4] ("action")
        n236 = event-data() -> ("CtlRef"=w314:refnum<vi>)  [unwired: 1 in]
        n237 = control-ref of="load"() -> (w317:refnum<vi>)
        n238 = control-ref of="format"() -> (w316:refnum<vi>)
        n239 = control-ref of="delete"() -> (w315:refnum<vi>)
        n240 = Unbundle By Name("usb") -> ("number in file name"=w308:u8)
        n241 = Build Array(w317, w316, w315) -> (w313:refnum<vi>[])
        n242 = Search 1D Array(1D array=w313, element=w314) -> (index of element=w306:i32)  [unwired: 1 in]
        n243 = local read "VGC"() -> (w312:refnum<class "PL Inficon VGC.lvclass">)
        n244 = Add(x=w307, y=w306) -> (x+y=w305:i32)
        n245 = call "USB Flash Drive Action.vi"("number in file name"=w308, "action"=w305, "VGC in"=w312) -> ("error out"=w310:errorcluster, "VGC out"=w311:refnum<class "PL Inficon VGC.lvclass">)  [unwired: 6 in, 1 out]
        n246 = local write "VGC"(w311) -> ()
        n247 = local write "error"(w310) -> ()
      }
      event "display settings.backlight, %": Value Change {
        n248 = event-data() -> ("NewVal"=w318:u8)  [unwired: 1 in]
        n249 = local read "VGC"() -> (w319:refnum<class "PL Inficon VGC.lvclass">)
        n250 = call "Configure Display Backlight.vi"("backlight, %"=w318, "VGC in"=w319) -> ("error out"=w320:errorcluster, "VGC out"=w321:refnum<class "PL Inficon VGC.lvclass">)  [unwired: 7 in, 1 out]
        n251 = local write "VGC"(w321) -> ()
        n252 = local write "error"(w320) -> ()
      }
      event "display settings.contrast, %": Value Change {
        n253 = event-data() -> ("NewVal"=w322:u8)  [unwired: 1 in]
        n254 = local read "VGC"() -> (w323:refnum<class "PL Inficon VGC.lvclass">)
        n255 = call "Configure Display Contrast.vi"("contrast, %"=w322, "VGC in"=w323) -> ("error out"=w324:errorcluster, "VGC out"=w325:refnum<class "PL Inficon VGC.lvclass">)  [unwired: 7 in, 1 out]
        n256 = local write "VGC"(w325) -> ()
        n257 = local write "error"(w324) -> ()
      }
      event "display settings.screensaver": Value Change {
        n258 = event-data() -> ("NewVal"=w326:u16)  [unwired: 1 in]
        n259 = local read "VGC"() -> (w327:refnum<class "PL Inficon VGC.lvclass">)
        n260 = call "Configure Display Screensaver.vi"("screensaver"=w326, "VGC in"=w327) -> ("error out"=w328:errorcluster, "VGC out"=w329:refnum<class "PL Inficon VGC.lvclass">)  [unwired: 7 in, 1 out]
        n261 = local write "VGC"(w329) -> ()
        n262 = local write "error"(w328) -> ()
      }
      event "display settings.language": Value Change {
        n263 = event-data() -> ("NewVal"=w330:u16)  [unwired: 1 in]
        n264 = local read "VGC"() -> (w331:refnum<class "PL Inficon VGC.lvclass">)
        n265 = call "Configure Display Language.vi"("language"=w330, "VGC in"=w331) -> ("error out"=w332:errorcluster, "VGC out"=w333:refnum<class "PL Inficon VGC.lvclass">)  [unwired: 7 in, 1 out]
        n266 = local write "VGC"(w333) -> ()
        n267 = local write "error"(w332) -> ()
      }
      event "display settings.number format": Value Change {
        n268 = event-data() -> ("NewVal"=w334:u16)  [unwired: 1 in]
        n269 = local read "VGC"() -> (w335:refnum<class "PL Inficon VGC.lvclass">)
        n270 = call "Configure Display Number Format.vi"("format"=w334, "VGC in"=w335) -> ("error out"=w336:errorcluster, "VGC out"=w337:refnum<class "PL Inficon VGC.lvclass">)  [unwired: 7 in, 1 out]
        n271 = local write "VGC"(w337) -> ()
        n272 = local write "error"(w336) -> ()
      }
      event "display settings.range": Value Change {
        n273 = event-data() -> ("NewVal"=w338:u16)  [unwired: 1 in]
        n274 = local read "VGC"() -> (w339:refnum<class "PL Inficon VGC.lvclass">)
        n275 = call "Configure Pressure Unit.vi"("unit"=w338, "VGC in"=w339) -> ("error out"=w340:errorcluster, "VGC out"=w341:refnum<class "PL Inficon VGC.lvclass">)  [unwired: 7 in, 1 out]
        n276 = local write "VGC"(w341) -> ()
        n277 = local write "error"(w340) -> ()
      }
      event "display settings.display resolutions": Value Change {
        n278 = event-data() -> ("NewVal"=w342:u16[])  [unwired: 1 in]
        n279 = local read "VGC"() -> (w343:refnum<class "PL Inficon VGC.lvclass">)
        n280 = call "Configure Display Resolutions.vi"("display resolutions"=w342, "VGC in"=w343) -> ("error out"=w344:errorcluster, "VGC out"=w345:refnum<class "PL Inficon VGC.lvclass">)  [unwired: 7 in, 1 out]
        n281 = local write "VGC"(w345) -> ()
        n282 = local write "error"(w344) -> ()
      }
      event "display settings.bar graph": Value Change {
        n283 = event-data() -> ("OldVal.channel"=w347:u16, "OldVal.graph mode"=w346:u16)  [unwired: 1 in]
        n284 = local read "VGC"() -> (w348:refnum<class "PL Inficon VGC.lvclass">)
        n285 = call "Configure Display Bar Graph.vi"("graph mode"=w346, "channel"=w347, "VGC in"=w348) -> ("error out"=w349:errorcluster, "VGC out"=w350:refnum<class "PL Inficon VGC.lvclass">)  [unwired: 5 in, 2 out]
        n286 = local write "VGC"(w350) -> ()
        n287 = local write "error"(w349) -> ()
      }
      event "communication settings.baud rate": Value Change {
        n288 = event-data() -> ("NewVal"=w351:u32)  [unwired: 1 in]
        n289 = local read "VGC"() -> (w354:refnum<class "PL Inficon VGC.lvclass">)
        n290 = call "Configure Baud Rate.vi"("baud rate"=w351, "VGC in"=w354) -> ("error out"=w352:errorcluster, "VGC out"=w353:refnum<class "PL Inficon VGC.lvclass">)  [unwired: 7 in, 1 out]
        n291 = property on="baud rate" class="Ring (strict)"("Value"=w351) -> ()  [unwired: 2 in, 2 out]
        n292 = local write "VGC"(w353) -> ()
        n293 = local write "error"(w352) -> ()
      }
      event "communication settings.ethernet": Value Change {
        w358 = u16 0 items=["disabled", "enabled"] ("dhcp")
        n294 = event-data() -> ("NewVal.dhcp"=w357:u32, "NewVal.ip address"=w355:string, "NewVal.subnet mask"=w360:string, "NewVal.default gateway"=w359:string)  [unwired: 1 in]
        n295 = local read "VGC"() -> (w363:refnum<class "PL Inficon VGC.lvclass">)
        n296 = Equal?(x=w357, y=w358) -> (x = y?=w356:bool)
        n297 = call "Configure Ethernet.vi"("default gateway"=w359, "subnet mask"=w360, "ip address"=w355, "dhcp"=w357, "VGC in"=w363) -> ("error out"=w361:errorcluster, "VGC out"=w362:refnum<class "PL Inficon VGC.lvclass">)  [unwired: 1 in, 4 out]
        n298 = case shown="True" w356 {
          tunnel: w355 -> [_ w364]
          frame False {
          }
          frame True {
            n299 = property on="ip address" class="Str"("Value"=w364) -> ()  [unwired: 2 in, 2 out]
          }
        }
        n300 = local write "VGC"(w362) -> ()
        n301 = local write "error"(w361) -> ()
      }
      event "reset errors": Value Change {
        n302 = event-data() -> ()  [unwired: 1 in, 6 out]
        n303 = local read "VGC"() -> (w374:refnum<class "PL Inficon VGC.lvclass">)
        n304 = call "Reset.vi"("VGC in"=w374) -> ("error out"=w372:errorcluster, "errors"=w371:u16[], "VGC out"=w373:refnum<class "PL Inficon VGC.lvclass">)  [unwired: 8 in]
        n305 = local write "VGC"(w373) -> ()
        n306 = local write "error"(w372) -> ()
        n307 = Array To Spreadsheet String(delimiter (Tab)=", ", array=w371, 3:"%d" ("format string")) -> (spreadsheet string=w368:string)
        n308 = call <vilib>:"Trim Whitespace.vi"("string"=w368) -> ("trimmed string"=w367:string)  [unwired: 1 in]
        n309 = Concatenate Strings("Errors: " ("string"), w367) -> (w365:string)
        n310 = One Button Dialog(message=w365) -> ()  [unwired: 1 in, 1 out]
      }
      event "error acknowledgement": Value Change {
        n311 = event-data() -> ("NewVal"=w375:u16)  [unwired: 1 in]
        n312 = local read "VGC"() -> (w378:refnum<class "PL Inficon VGC.lvclass">)
        n313 = call "Configure Error Acknowledgement.vi"("error acknowledgement"=w375, "VGC in"=w378) -> ("error out"=w376:errorcluster, "VGC out"=w377:refnum<class "PL Inficon VGC.lvclass">)  [unwired: 7 in, 1 out]
        n314 = local write "VGC"(w377) -> ()
        n315 = local write "error"(w376) -> ()
      }
      event "save parameters": Value Change {
        n316 = event-data() -> ()  [unwired: 1 in, 6 out]
        n317 = local read "VGC"() -> (w382:refnum<class "PL Inficon VGC.lvclass">)
        n318 = call "Save Parameters to EEPROM.vi"("parameters"="parameters", "VGC in"=w382) -> ("error out"=w380:errorcluster, "VGC out"=w381:refnum<class "PL Inficon VGC.lvclass">)  [unwired: 8 in]
        n319 = local write "VGC"(w381) -> ()
        n320 = local write "error"(w380) -> ()
      }
      event "continuous measurement": Value Change {
        n321 = event-data() -> ("NewVal"=w383:bool)  [unwired: 1 in]
        "continuous read" <- w383
        n322 = case shown="True" w383 {
          frame False {
          }
          frame True {
            n323 = local read "VGC"() -> (w391:refnum<class "PL Inficon VGC.lvclass">)
            n324 = case shown="2" "continuous time interval" {
              tunnel: [0.1 1.0 60.0] -> w386
              frame 0, Default {
              }
              frame 1 {
              }
              frame 2 {
              }
            }
            n325 = call "Start Continuous Output.vi"("time interval (1 s)"="continuous time interval", "VGC in"=w391) -> ("error out"=w389:errorcluster, "VGC out"=w390:refnum<class "PL Inficon VGC.lvclass">)  [unwired: 8 in]
            n326 = Bundle(0.0, w386, dbl[][] []) -> (w384:cluster{dbl, dbl, dbl[][]})  [unwired: 1 in]
            n327 = local write "VGC"(w390) -> ()
            n328 = local write "error"(w389) -> ()
            n329 = local write "continuous measurement graph"(w384) -> ()
          }
        }
      }
      event "test ADC": Value Change {
        n330 = event-data() -> ()  [unwired: 1 in, 1 out]
        n331 = local read "VGC"() -> (w402:refnum<class "PL Inficon VGC.lvclass">)
        n332 = call "Test ADC.vi"("VGC in"=w402) -> ("error out"=w400:errorcluster, "measured signals, V"=w397:dbl[], "VGC out"=w401:refnum<class "PL Inficon VGC.lvclass">)  [unwired: 8 in]
        n333 = local write "VGC"(w401) -> ()
        n334 = local write "error"(w400) -> ()
        n335 = Array To Spreadsheet String(delimiter (Tab)=", ", array=w397, 3:"%#g V" ("format string")) -> (spreadsheet string=w396:string)
        n336 = call <vilib>:"Trim Whitespace.vi"("string"=w396) -> ("trimmed string"=w395:string)  [unwired: 1 in]
        n337 = One Button Dialog(message=w395) -> ()  [unwired: 1 in, 1 out]
      }
      event "test ID resistance": Value Change {
        n338 = event-data() -> ()  [unwired: 1 in, 1 out]
        n339 = local read "VGC"() -> (w410:refnum<class "PL Inficon VGC.lvclass">)
        n340 = call "Test ID Resistance.vi"("VGC in"=w410) -> ("error out"=w408:errorcluster, "ID resistance, kOhm"=w405:dbl[], "VGC out"=w409:refnum<class "PL Inficon VGC.lvclass">)  [unwired: 8 in]
        n341 = local write "VGC"(w409) -> ()
        n342 = local write "error"(w408) -> ()
        n343 = Array To Spreadsheet String(delimiter (Tab)=", ", array=w405, 3:"%#g kOhm" ("format string")) -> (spreadsheet string=w404:string)
        n344 = call <vilib>:"Trim Whitespace.vi"("string"=w404) -> ("trimmed string"=w403:string)  [unwired: 1 in]
        n345 = One Button Dialog(message=w403) -> ()  [unwired: 1 in, 1 out]
      }
      event "test display": Value Change {
        w413 = u16 0 items=["off", "on"] ("state")
        w414 = u16 1 items=["off", "on"] ("state")
        n346 = event-data() -> ("NewVal"=w412:bool)  [unwired: 1 in]
        n347 = local read "VGC"() -> (w417:refnum<class "PL Inficon VGC.lvclass">)
        n348 = Select(t=w414, s=w412, f=w413) -> (s? t:f=w411:u16)
        n349 = call "Test Display.vi"("state"=w411, "VGC in"=w417) -> ("error out"=w415:errorcluster, "VGC out"=w416:refnum<class "PL Inficon VGC.lvclass">)  [unwired: 7 in, 1 out]
        n350 = local write "VGC"(w416) -> ()
        n351 = local write "error"(w415) -> ()
      }
      event "test EEPROM": Value Change {
        n352 = event-data() -> ()  [unwired: 1 in, 1 out]
        n353 = local read "VGC"() -> (w423:refnum<class "PL Inficon VGC.lvclass">)
        n354 = call "Test EEPROM.vi"("VGC in"=w423) -> ("error out"=w421:errorcluster, "error word"=w418:u16, "VGC out"=w422:refnum<class "PL Inficon VGC.lvclass">)  [unwired: 8 in]
        n355 = local write "VGC"(w422) -> ()
        n356 = local write "error"(w421) -> ()
        n357 = Format Into String(format string="Error word: 0x%x", w418) -> (resulting string=w419:string)  [unwired: 2 in, 1 out]
        n358 = One Button Dialog(message=w419) -> ()  [unwired: 1 in, 1 out]
      }
      event "test flash": Value Change {
        n359 = event-data() -> ()  [unwired: 1 in, 1 out]
        n360 = local read "VGC"() -> (w430:refnum<class "PL Inficon VGC.lvclass">)
        n361 = call "Test Flash.vi"("VGC in"=w430) -> ("error out"=w428:errorcluster, "checksum"=w424:u32, "error word"=w425:u16, "VGC out"=w429:refnum<class "PL Inficon VGC.lvclass">)  [unwired: 7 in]
        n362 = local write "VGC"(w429) -> ()
        n363 = local write "error"(w428) -> ()
        n364 = Format Into String(format string="Error word: 0x%x. Checksum: 0x%x.", w425, w424) -> (resulting string=w426:string)  [unwired: 2 in, 1 out]
        n365 = One Button Dialog(message=w426) -> ()  [unwired: 1 in, 1 out]
      }
      event "test relays": Value Change {
        w435 = u16 0 items=["off", "on"] ("state")
        n366 = event-data() -> ()  [unwired: 1 in, 1 out]
        n367 = local read "VGC"() -> (w440:refnum<class "PL Inficon VGC.lvclass">)
        n368 = for {
          N: 7 -> [_]
          tunnel: [w447] -> w438
          shift-right: [w446] -> w439
          shift-left: w440 -> [w458]
          tunnel: [FALSE ("test relays")] -> w434
          i -> [w454]
          stop <- w448 stop-if-true
          w456 = u16 1 items=["off", "on"] ("state")
          n369 = Logical Shift(y=w454, x=u16 1) -> (x << y=w453:u16)
          n370 = Number To Boolean Array(number=w453) -> (Boolean array=w452:bool[])
          n371 = Array To Cluster(array=w452) -> (cluster=w451:T13)
          n372 = Wait (ms)(milliseconds to wait=u32 1000) -> ()  [unwired: 1 out]
          n373 = call "Test Relays.vi"("relays"=w451, "state"=w456, "VGC in"=w458) -> ("error out"=w448:errorcluster, "VGC out"=w449:refnum<class "PL Inficon VGC.lvclass">)  [unwired: 5 in, 2 out]
          n374 = call "Read Relay Test State.vi"("error in (no error)"=w448, "VGC in"=w449) -> ("error out"=w447:errorcluster, "relays"=w444:T11, "state"=→"relay test state":u16, "VGC out"=w446:refnum<class "PL Inficon VGC.lvclass">)  [unwired: 6 in]
          n375 = Cluster To Array(cluster=w444) -> (array=→"relay test relays":bool[])
        }
        n376 = local write "test relays"(w434) -> ()
        n377 = call "Test Relays.vi"("error in (no error)"=w438, "relays"=T11 {"switching function relay 1"=FALSE, "switching function relay 2"=FALSE, "switching function relay 3"=FALSE, "switching function relay 4"=FALSE, "switching function relay 5"=FALSE, "switching function relay 6"=FALSE, "error relay"=FALSE}, "state"=w435, "VGC in"=w439) -> ("error out"=w441:errorcluster, "relays"=w431:T11, "state"=w433:u16, "VGC out"=w442:refnum<class "PL Inficon VGC.lvclass">)  [unwired: 4 in]
        n378 = local write "relay test state"(w433) -> ()
        n379 = local write "VGC"(w442) -> ()
        n380 = local write "error"(w441) -> ()
        n381 = Cluster To Array(cluster=w431) -> (array=w432:bool[])
        n382 = local write "relay test relays"(w432) -> ()
      }
      event "test keys": Value Change {
        n383 = event-data() -> ()  [unwired: 1 in, 1 out]
        n384 = local read "VGC"() -> (w466:refnum<class "PL Inficon VGC.lvclass">)
        n385 = call "Test Keys.vi"("VGC in"=w466) -> ("error out"=w467:errorcluster, "keys"=w462:T14, "VGC out"=w468:refnum<class "PL Inficon VGC.lvclass">)  [unwired: 8 in]
        n386 = Cluster To Array(cluster=w462) -> (array=w461:u16[])
        n387 = local write "VGC"(w468) -> ()
        n388 = local write "error"(w467) -> ()
        n389 = for {
          tunnel: w461 -> [w477] mode=indexing
          tunnel: [w470] -> w460 mode=indexing
          i -> [w472]
          w476 = u16 1 items=["not pushed", "pushed"] ("key 3")
          n390 = Equal?(x=w477, y=w476) -> (x = y?=w475:bool)
          n391 = Increment(x=w472) -> (x+1=w471:i32)
          n392 = Select(t="pushed" ("format string"), s=w475, f="not pushed" ("format string")) -> (s? t:f=w469:string)
          n393 = Format Into String(format string="Key %d: %s.", w471, w469) -> (resulting string=w470:string)  [unwired: 2 in, 1 out]
        }
        n394 = call <vilib>:"Space Constant.vi"() -> ("String"=w459:string)
        n395 = Array To Spreadsheet String(delimiter (Tab)=w459, array=w460, 3:"%s" ("format string")) -> (spreadsheet string=w464:string)
        n396 = call <vilib>:"Trim Whitespace.vi"("string"=w464) -> ("trimmed string"=w463:string)  [unwired: 1 in]
        n397 = One Button Dialog(message=w463) -> ()  [unwired: 1 in, 1 out]
      }
      event "interface", "TCP settings", "serial settings": Value Change {
        n398 = event-data() -> ()  [unwired: 1 in, 1 out]
        n399 = local read "VGC"() -> (w484:refnum<class "PL Inficon VGC.lvclass">)
        n400 = call "Close.vi"("VGC in"=w484) -> ("error out"=w483:errorcluster)  [unwired: 10 in]
        n401 = call <vilib>:"Clear Errors.vi"("error in (no error)"=w483) -> ("error out"=w481:errorcluster)  [unwired: 5 in, 1 out]
        n402 = case shown="\"TCP\"" "interface" {
          tunnel: w481 -> [w490 w491]
          tunnel: [w486 w495] -> w480
          tunnel: [w485 w494] -> w479
          frame "serial", Default {
            n403 = Unbundle By Name("serial settings") -> ("port"=w488:refnum<visa-resource-name>, "baud rate"=w487:u32)
            n404 = call "Initialize Serial.vi"("error in (no error)"=w490, "baud rate (115200)"=w487, "port"=w488) -> ("error out"=w485:errorcluster, "VGC out"=w486:refnum<class "PL Inficon VGC.lvclass">)  [unwired: 7 in]
          }
          frame "TCP" {
            n405 = Unbundle By Name("TCP settings") -> ("ip address"=w493:string, "port"=w492:u16)
            n406 = call "Initialize TCP.vi"("error in (no error)"=w491, "port (8000)"=w492, "ip address"=w493) -> ("error out"=w494:errorcluster, "VGC out"=w495:refnum<class "PL Inficon VGC.lvclass">)  [unwired: 7 in]
          }
        }
        "error" <- w479
        "VGC" <- w480
      }
      event "error": Mouse Up {
        n407 = event-data() -> ()  [unwired: 1 in, 1 out]
        n408 = local read "error"() -> (w497:errorcluster)
        n409 = call <vilib>:"Simple Error Handler.vi"("error in (no error)"=w497) -> ()  [unwired: 4 in, 5 out]
      }
      event "stop": Value Change {
        n410 = event-data() -> ()  [unwired: 1 in, 1 out]
        n411 = local read "VGC"() -> (w499:refnum<class "PL Inficon VGC.lvclass">)
        n412 = call "Close.vi"("VGC in"=w499) -> ("error out"=w498:errorcluster)  [unwired: 10 in]
        n413 = call <vilib>:"Clear Errors.vi"("error in (no error)"=w498) -> ()  [unwired: 5 in, 2 out]
      }
    }
  }
